vi "receiveData.vi"(8 "error in (no error)":errorcluster, 11 "Model in":refnum<class "Model.lvclass">) -> (0 "error out":errorcluster, 3 "Model out":refnum<class "Model.lvclass">)   [LabVIEW 2016, in "Model.lvclass"]
uses:
  Model.lvclass
  Model.lvclass/Model.ctl
  Common_ILC/ILC/ILC.lvclass
  UserEvents/UserEvents.lvclass
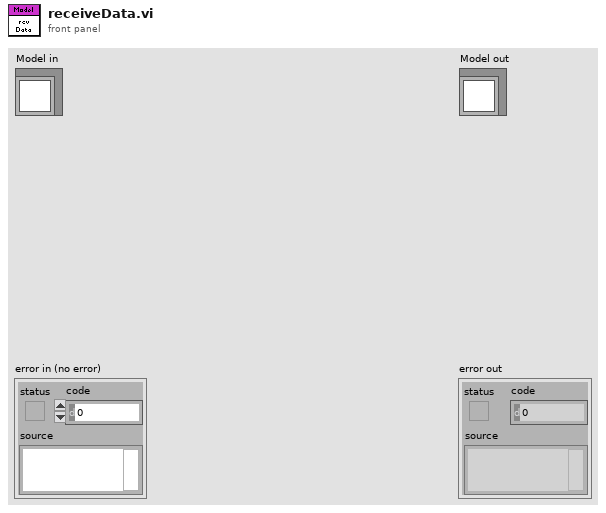
[diagram p1: front panel]
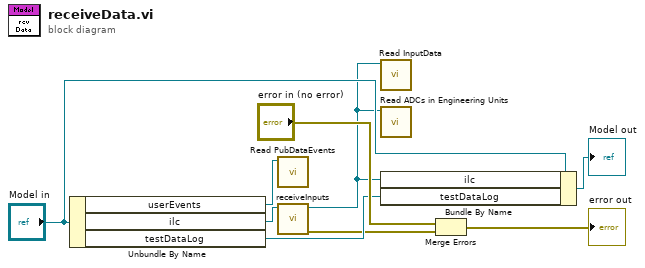
[diagram p0: block diagram]
diagram:
  n1 = Unbundle By Name("Model in") -> ("userEvents"=w5:refnum<class "UserEvents.lvclass">, "ilc"=w4:refnum<class "ILC.lvclass">, "testDataLog"=w3:refnum<class "TestDataLog.lvclass">)
  n2 = call "Read PubDataEvents.vi"("UserEvents in"=w5) -> ()  [unwired: 9 in, 2 out]
  n3 = call "receiveInputs.vi"("ILC in"=w4) -> ("error out"=w1:errorcluster, "ILC out"=w2:refnum<class "ILC.lvclass">)  [unwired: 7 in, 2 out]
  n4 = call "Read InputData.vi"("ILC in"=w2) -> ()  [unwired: 9 in, 2 out]
  n5 = call "Read ADCs in Engineering Units.vi"("ILC in"=w2) -> ()  [unwired: 9 in, 2 out]
  n6 = Bundle By Name(cluster="Model in", "ilc"=w2, "testDataLog"=w3) -> (→"Model out":refnum<class "Model.lvclass">)
  n7 = Merge Errors("error in (no error)", w1) -> (→"error out":errorcluster)
